vi "Is Data Modified.vi"(8 "error in (no error)":errorcluster) -> (0 "error out":errorcluster, 3 "Data Modified?":bool)   [LabVIEW 2014, in "Map Data.lvlib"]
doc: "Returns if there have been changes made to the address book data store since the last save."
uses:
  Map Data.lvlib
  MapCommand.ctl
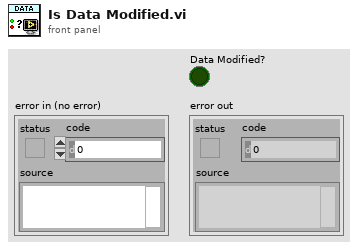
[diagram p1: front panel]
types:
  T1 = typedef "Map Data.lvlib/MapCommand.ctl" = enum16{"Load", "Update Cursor", "Save", "Get All Data", "Get Single Data", "Set Single Data", "Delete All", "Remove Single Data", "Set Favorite Status", "Is Data Modified", "Import Data"}
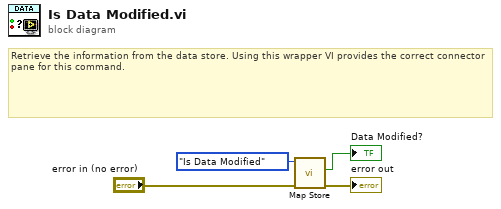
[diagram p0: block diagram]
diagram:
  # "Retrieve the information from the data store. Using this wrapper VI provides the correct connector pane for this command."
  n1 = call "Map Store.vi"("error in (no error)"="error in (no error)", "Command"=MapCommand."Is Data Modified") -> ("error out"=→"error out":errorcluster, "Data Modified?"=→"Data Modified?":bool)  [unwired: 6 in, 2 out]
